vi "GetHistoricalMinMax.vi"(7 "LabVIEW Web Service Request":refnum<class "Web Request.lvclass">) -> ()   [LabVIEW 2014]
uses:
  <vilib>/wsapi/Web Request.lvclass
  IndoorData_class/HistoricalMinMax.ctl
  PI_WeatherStation/WebServiceData_class/WebServiceData.lvclass
  IndoorData_class/IndoorData.lvclass
panel:
  # "Use the Web Service Request input terminal to call the VIs on the Web Services palette. Do not remove it from the connector pane unless you don't need access to the palette."
  # "Each additional control wired to the connector pane will be available as an input in the URL. To include an indicator in terminal-mode output (the default setting), it must also be wired to the connector pane."
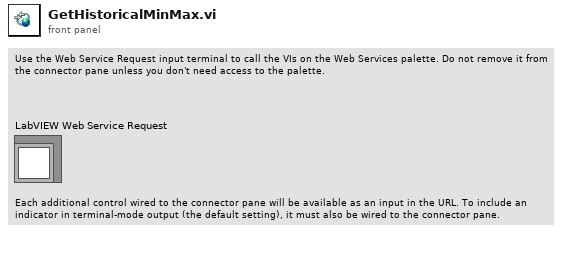
[diagram p1: front panel]
types:
  T1 = typedef "IndoorData.lvclass/HistoricalMinMax.ctl" = cluster{"Time":dbl[], "Temp Max":dbl[], "Temp Min":dbl[], "RH Max":dbl[], "RH Min":dbl[]}
  T2 = typedef "WebServiceData.lvclass/BufferType.ctl" = cluster{"Time":dbl[], "Temp":dbl[], "RH":dbl[]}
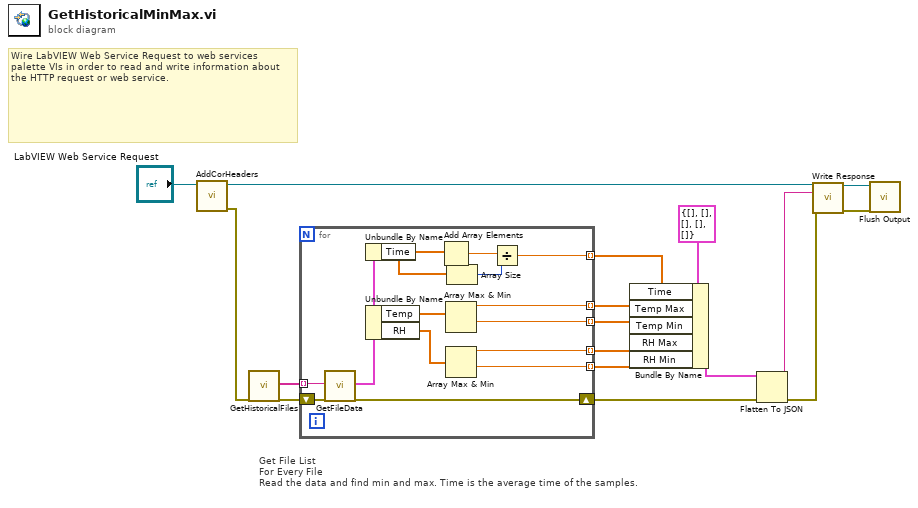
[diagram p0: block diagram]
diagram:
  # "Get File List\nFor Every File\nRead the data and find min and max. Time is the average time of the samples."
  # "Wire LabVIEW Web Service Request to web services palette VIs in order to read and write information about the HTTP request or web service."
  n1 = call "AddCorHeaders.vi"("LabVIEW Web Service Request"="LabVIEW Web Service Request") -> ("error out"=w10:errorcluster, "LabVIEW Web Service Request out"=w14:refnum<class "Web Request.lvclass">)  [unwired: 9 in]
  n2 = call "GetHistoricalFiles.vi"("error in (no error)"=w10) -> ("filenames"=w8:string[], "error out"=w9:errorcluster)  [unwired: 17 in]
  n3 = for {
    shift-right: [w31] -> w17
    shift-left: w9 -> [w30]
    tunnel: w8 -> [w29] mode=indexing
    tunnel: [w26] -> w5 mode=indexing
    tunnel: [w25] -> w6 mode=indexing
    tunnel: [w23] -> w3 mode=indexing
    tunnel: [w22] -> w4 mode=indexing
    tunnel: [w18] -> w2 mode=indexing
    n4 = call "GetFileData.vi"("Filename"=w29, "error in (no error)"=w30) -> ("HourlyAVGBuffer"=w28:T2, "error out"=w31:errorcluster)  [unwired: 16 in]
    n5 = Unbundle By Name(w28) -> ("Time"=w21:dbl[])
    n6 = Unbundle By Name(w28) -> ("Temp"=w24:dbl[], "RH"=w27:dbl[])
    n7 = Add Array Elements(numeric array=w21) -> (sum=w20:dbl)
    n8 = Array Max & Min(array=w24) -> (max value=w23:dbl, min value=w22:dbl)  [unwired: 2 out]
    n9 = Array Max & Min(array=w27) -> (max value=w26:dbl, min value=w25:dbl)  [unwired: 2 out]
    n10 = Array Size(array=w21) -> (size(s)=w19:i32)
    n11 = Divide(x=w20, y=w19) -> (x/y=w18:dbl)
  }
  n12 = Bundle By Name(cluster=T1 {"Time"=[], "Temp Max"=[], "Temp Min"=[], "RH Max"=[], "RH Min"=[]}, "Time"=w2, "Temp Max"=w3, "Temp Min"=w4, "RH Max"=w5, "RH Min"=w6) -> (w1:T1)
  n13 = Flatten To JSON(anything=w1, error in (no error)=w17) -> (JSON string=w12:string, 11:w13:errorcluster)  [unwired: 1 in]
  n14 = call <vilib>:"Write Response.vi"("LabVIEW Web Service Request"=w14, "response string"=w12, "error in (no error)"=w13) -> ("LabVIEW Web Service Request out"=w16:refnum<class "Web Request.lvclass">, "error out"=w15:errorcluster)  [unwired: 11 in]
  n15 = call <vilib>:"Flush Output.vi"("LabVIEW Web Service Request"=w16, "error in (no error)"=w15) -> ()  [unwired: 12 in, 2 out]
